vi "File_CleanClose.vi"(8 "error in (no error)":errorcluster, 11 "File in":refnum<class "File.lvclass">) -> (0 "error out":errorcluster, 2 "old path":path, 3 "File out":refnum<class "File.lvclass">)   [LabVIEW 2024, in "File.lvclass"]
doc: "Closes the file and defragments the resulting TDMS file to preserve space."
uses:
  File.lvclass
  File.lvclass/File.ctl
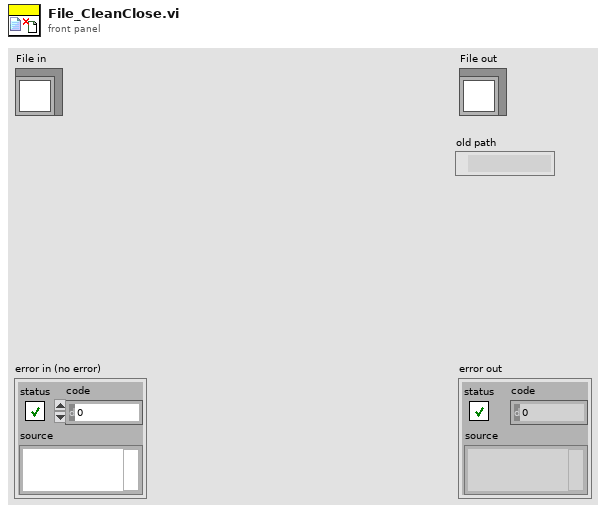
[diagram p1: front panel]
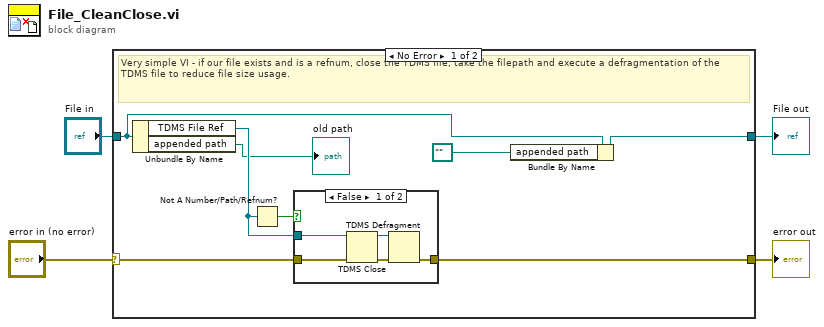
[diagram p0: block diagram]
diagram:
  n1 = case shown="No Error" "error in (no error)" {
    selector: "error in (no error)" -> [w12 w20]
    tunnel: [w11 w20] -> w3
    tunnel: [w6 w19] -> w1
    tunnel: "File in" -> [w10 w19]
    frame No Error {
      # "Very simple VI - if our file exists and is a refnum, close the TDMS file, take the filepath and execute a defragmentation of the TDMS file to reduce file size usage."
      n2 = Unbundle By Name(w10) -> ("TDMS File Ref"=w8:refnum<k34>, "appended path"=→"old path":path)
      n3 = Not A Number/Path/Refnum?(number/path/refnum=w8) -> (NaN/Path/Refnum?=w9:bool)
      n4 = case shown="False" w9 {
        tunnel: w12 -> [w16 w18]
        tunnel: [w15 w18] -> w11
        tunnel: w8 -> [w13 _]
        frame False {
          n5 = TDMS Close(8:w16, 11:w13) -> (0:w17:errorcluster, 3:w14:path)
          n6 = TDMS Defragment(4:w17, 7:w14) -> (0:w15:errorcluster)
        }
        frame True {
        }
      }
      n7 = Bundle By Name(cluster=w10, "appended path"=path "") -> (w6:refnum<class "File.lvclass">)
    }
    frame Error {
    }
  }
  "error out" <- w3
  "File out" <- w1
